vi "Destructor.vi"(8 "error in (no error)":errorcluster, 11 "INL Valve Controller in":refnum<class "INL Valve Controller.lvclass">) -> (0 "error out":errorcluster, 3 "INL Valve Controller out":refnum<class "INL Valve Controller.lvclass">)   [LabVIEW 2011, in "INL Valve Controller.lvclass"]
uses:
  INL Valve Controller.lvclass
  Valve Controller/Status.ctl
  Valve Controller/Valves.ctl
  INL Valve Controller.lvclass/INL Valve Controller.ctl
  Valve Controller/Valve Controller.lvclass
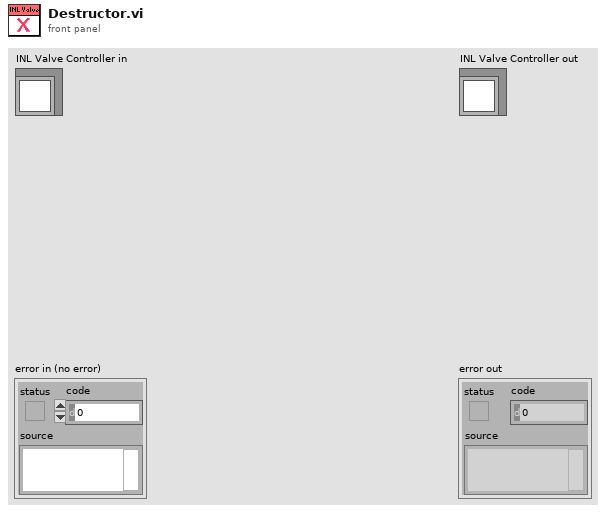
[diagram p1: front panel]
types:
  T1 = typedef "Valve Controller.lvclass/Status.ctl" = u16
  T2 = typedef "Valve Controller.lvclass/Valves.ctl" = u16
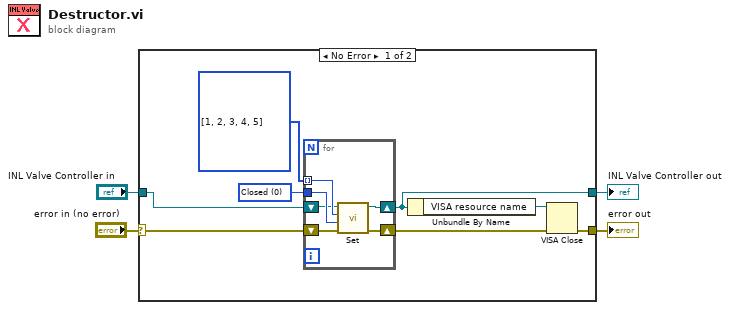
[diagram p0: block diagram]
diagram:
  n1 = case shown="No Error" "error in (no error)" {
    selector: "error in (no error)" -> [w5 w20]
    tunnel: [w7 w20] -> w3
    tunnel: [w6 w19] -> w1
    tunnel: "INL Valve Controller in" -> [w9 w19]
    frame No Error {
      w11 = T1 0 items=["Closed", "Open"] ("status in")
      w12 = T2[] [1, 2, 3, 4, 5] items=["Valve 1"=1, "Valve 2"=2, "Valve 3"=3, "Valve 4"=4, "Valve 5"=5, "Valve 6"=6, "Valve 7"=7]
      n2 = for {
        tunnel: w12 -> [w14] mode=indexing
        tunnel: w11 -> [w17]
        shift-right: [w16] -> w6
        shift-left: w9 -> [w13]
        shift-right: [w15] -> w10
        shift-left: w5 -> [w18]
        n3 = call-dynamic "Set.vi"("error in (no error)"=w18, "status in"=w17, "valve in"=w14, "INL Valve Controller in"=w13) -> ("error out"=w15:errorcluster, "INL Valve Controller out"=w16:refnum<class "INL Valve Controller.lvclass">)  [unwired: 4 in, 2 out]
      }
      n4 = Unbundle By Name(w6) -> ("VISA resource name"=w8:refnum<visa-resource-name>)
      n5 = VISA Close(VISA resource name=w8, error in (no error)=w10) -> (error out=w7:errorcluster)
    }
    frame Error {
    }
  }
  "error out" <- w3
  "INL Valve Controller out" <- w1
